vi "GUI_Windmill.vi"() -> ()   [LabVIEW 2020]
uses:
  Device Drivers/TapeDrive/Direction_TypDef.ctl
  Shared/Device Driver/OnOffTypeDef.ctl
  Shared/GUI_Template/GUI_master/tcp new data cluster.ctl
panel:
  out "error out":errorcluster
  in  "position::1":dbl=5.0 caption="Position" min=0.0 max=9999999999.0
  in  "MinMonMaxCounts::1":dbl=5.0 caption="MinCountsMax" min=0.0 max=5000.0
  in  "MinMonMeanCountsRaw::1":dbl=5.0 caption="Min mean" min=0.0 max=5000.0
  in  "AutoStep::1":T1 caption="AutoStep"
  in  "MotorDirection::1":T2 caption="Direction"
  in  "GUIdevice 1":string="WIND-PL1-STAGE1"
  in  "step::1":bool caption="Move Tape"
  in  "stop":bool
  # "Windmill"
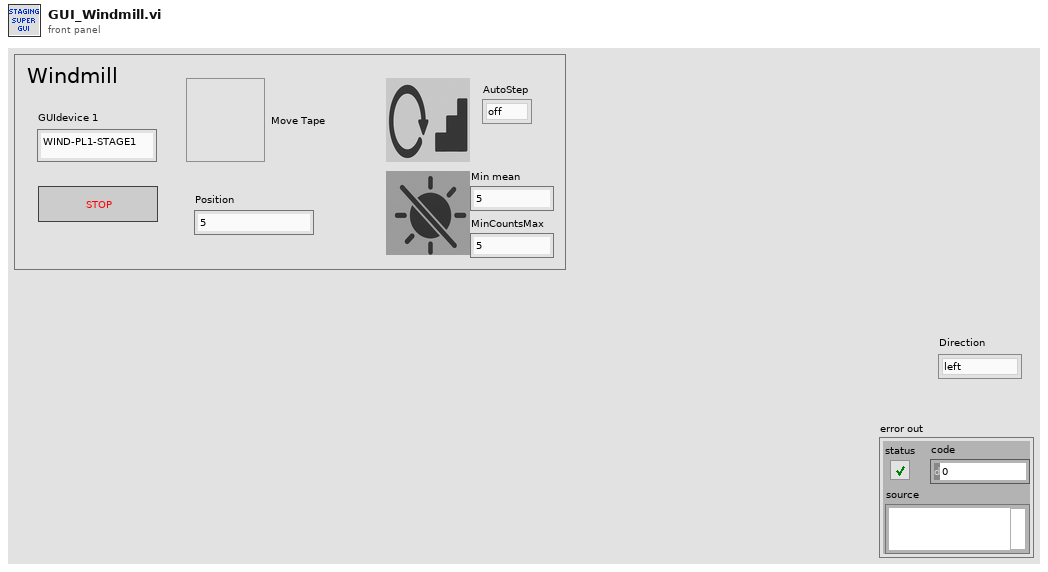
[diagram p1: front panel]
types:
  T1 = typedef "OnOffTypeDef.ctl" = enum16{"off", "on"}
  T2 = typedef "Direction_TypDef.ctl" = enum16{"left", "right"}
  T3 = enum32{"invalid app kind", "Development System", "Run Time System", "Student Edition", "Embedded LabVIEW", "Evaluation", "Custom"}
  T4 = typedef "tcp new data cluster.ctl" = cluster{"EventEnum":enum16{"new data", "connection status update"}, "Device name":string}
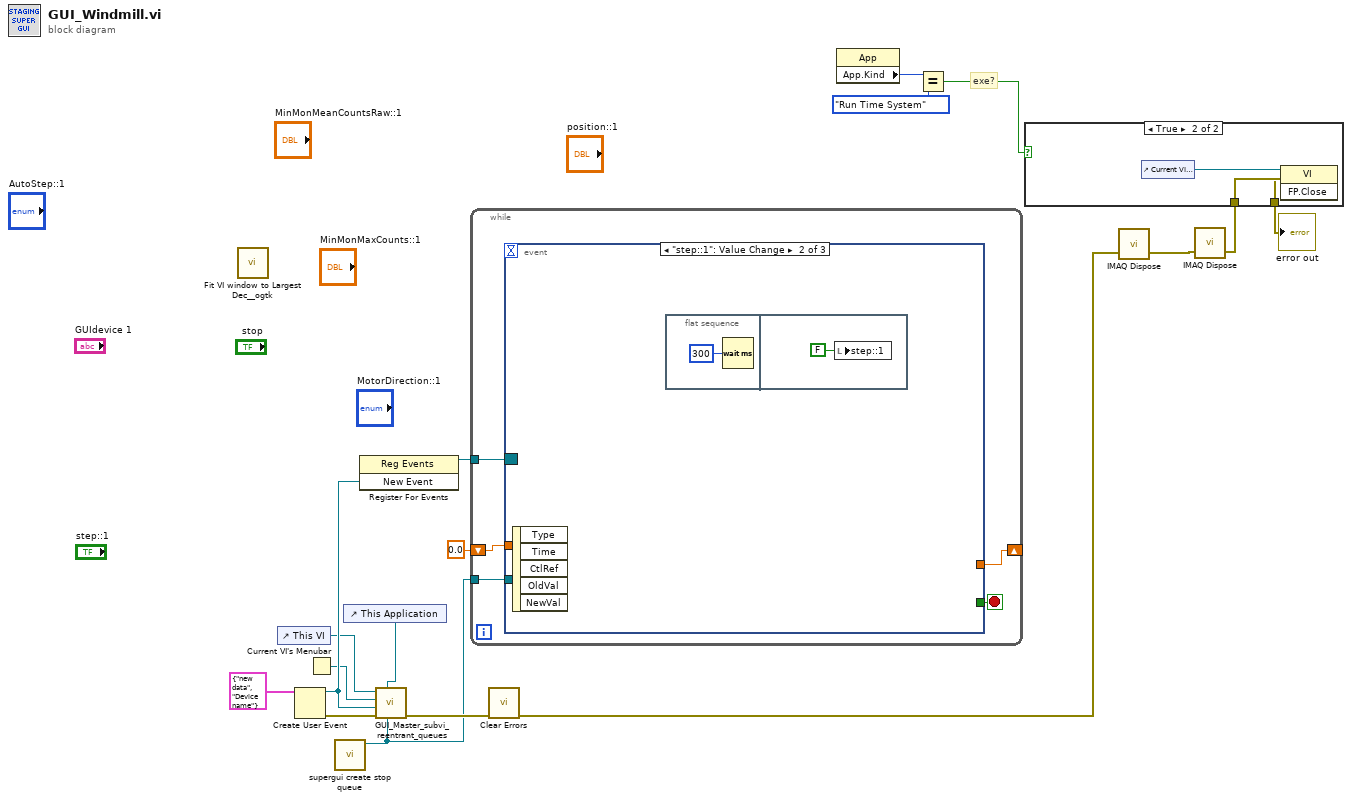
[diagram p0: block diagram]
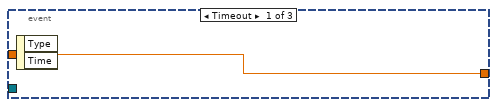
[diagram p3: hidden frame]
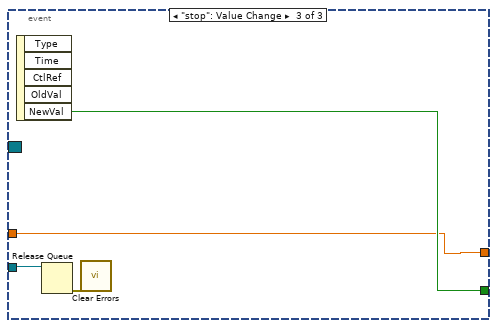
[diagram p4: hidden frame]
diagram:
  # "exe?"
  n1 = call <userlib>:"Fit VI window to Largest Dec__ogtk.vi"() -> ()  [unwired: 6 in, 2 out]
  n2 = control-ref of="This VI"() -> (w9:refnum<vi>)
  n3 = Create User Event(user event datatype=T4 {"EventEnum"=enum."new data", "Device name"="Device name"} ("New Event")) -> (user event=w14:refnum<user-event>, error out=w16:errorcluster)  [unwired: 1 in]
  n4 = Current VI's Menubar() -> (w8:refnum<k9>)
  n5 = call "supergui create stop queue.vi"() -> ("STOP Queue out"=w6:refnum<queue>)  [unwired: 11 in]
  n6 = control-ref of="This Application"() -> (w7:refnum<vi>)
  n7 = register-events(w14) -> (reference out=w13:refnum<event-registration>)  [unwired: 2 in, 1 out]
  n8 = call "GUI_Master_subvi_reentrant_queues.vi"("STOP Queue in"=w6, "This Application"=w7, "error in (no error)"=w16, "tcp data event"=w14, "Caller menu reference"=w8, "Caller VI ref"=w9) -> ("error out"=w15:errorcluster)  [unwired: 5 in]
  n9 = while {
    tunnel: w13 -> [w22]
    shift-right: [w19] -> _
    shift-left: 0.0 -> [w20]
    tunnel: w6 -> [w18]
    stop <- w21 stop-if-true
    n10 = event shown="[1] \"step::1\": Value Change" {
      selector: w22 -> [_ _ _]
      dyn-events: _ -> [_ _ _]
      timeout: _ -> [_ _ _]
      tunnel: [_ _ w29] -> w21
      tunnel: w20 -> [w23 _ w28]
      tunnel: [w23 _ w28] -> w19
      tunnel: w18 -> [_ _ w27]
      event Timeout {
        n11 = event-data() -> ()  [unwired: 1 in, 2 out]
      }
      event "step::1": Value Change {
        n12 = event-data() -> ()  [unwired: 1 in, 5 out]
        n13 = flat-sequence {
          frame #0 {
            n14 = Wait (ms)(milliseconds to wait=u32 300) -> ()  [unwired: 1 out]
          }
          frame #1 {
            n15 = local write "step::1"(FALSE ("Step::1")) -> ()
          }
        }
      }
      event "stop": Value Change {
        n16 = event-data() -> ("NewVal"=w29:bool)  [unwired: 1 in, 4 out]
        n17 = Release Queue(queue=w27) -> (error out=w26:errorcluster)  [unwired: 2 in, 2 out]
        n18 = call <vilib>:"Clear Errors.vi"("error in (no error)"=w26) -> ()  [unwired: 5 in, 2 out]
      }
    }
  }
  n19 = call <vilib>:"Clear Errors.vi"("error in (no error)"=w15) -> ("error out"=w11:errorcluster)  [unwired: 5 in, 1 out]
  n20 = property class="App"() -> ("App.Kind"=w4:T3)  [unwired: 2 in, 2 out]
  n21 = Equal?(x=w4, y=T3."Run Time System" ("Application:Kind")) -> (x = y?=w2:bool)
  n22 = call "IMAQ Dispose"("error in (no error)"=w11) -> ("error out"=w10:errorcluster)  [unwired: 5 in]
  n23 = call "IMAQ Dispose"("error in (no error)"=w10) -> ("error out"=w5:errorcluster)  [unwired: 5 in]
  n24 = case shown="True" w2 {
    tunnel: w5 -> [w30 w33]
    tunnel: [w30 w31] -> w1
    frame False {
    }
    frame True {
      n25 = control-ref of="Current VI Reference"() -> (w32:refnum<vi>)
      n26 = invoke class="VI" method="FP.Close"(reference=w32, error in=w33) -> (error out=w31:errorcluster)  [unwired: 1 in, 2 out]
    }
  }
  "error out" <- w1
